vi "_computeInput.vi"(10 "HistoryYUR":dbl[][][](array[numeric]), 11 "Coeff.RST":dbl[][][](array[numeric])) -> (3 "u":dbl[](array[numeric]))   [LabVIEW 2021, in "System.lvclass"]
uses:
  System.lvclass
  <vilib>/Analysis/baseanly.llb/Real Dot Product.vi
  System.lvclass/System.ctl
  <vilib>/Analysis/NI_AALBase.lvlib
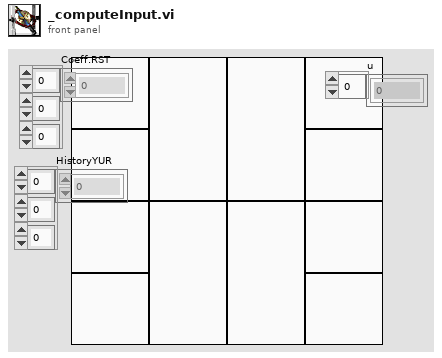
[diagram p1: front panel]
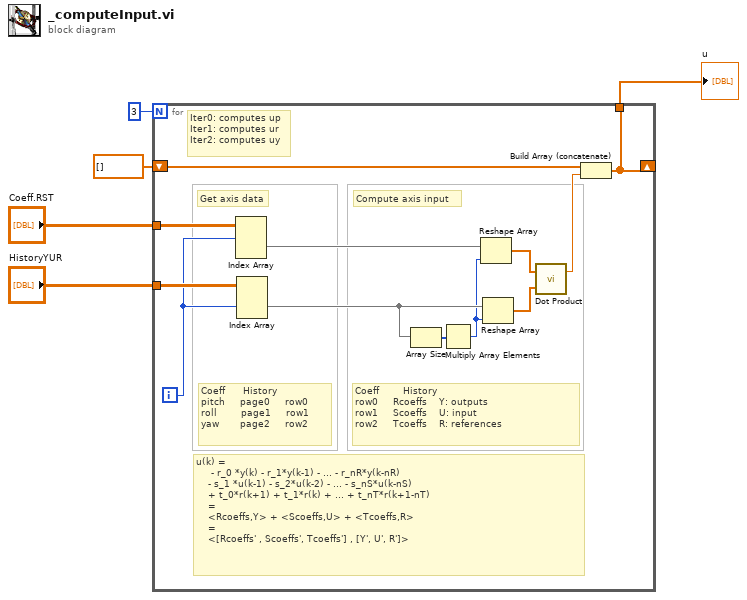
[diagram p0: block diagram]
diagram:
  n1 = for {
    N: 3 -> [_]
    tunnel: "Coeff.RST" -> [w17]
    tunnel: "HistoryYUR" -> [w16]
    shift-right: [w7] -> _
    shift-left: dbl[] [] -> [w8]
    tunnel: [w7] -> w5
    i -> [w6]
    # "u(k) = \n     - r_0 *y(k) - r_1*y(k-1) - ... - r_nR*y(k-nR) \n    - s_1 *u(k-1) - s_2*u(k-2) - ... - s_nS*u(k-nS) \n    + t_0*r(k+1) + t_1*r(k) + ... + t_nT*r(k+1-nT)\n    =\n    <Rcoeffs,Y> + <Scoeffs,U> + <Tcoeffs,R>\n    = \n    <[Rcoeffs' , Scoeffs', Tcoeffs'] , [Y', U', R']>"
    # "Iter0: computes up\nIter1: computes ur\nIter2: computes uy"
    # "Compute axis input"
    # "Coeff        History\nrow0     Rcoeffs    Y: outputs\nrow1     Scoeffs    U: input\nrow2     Tcoeffs    R: references"
    # "Get axis data"
    # "Coeff      History\npitch     page0     row0\nroll        page1     row1\nyaw       page2     row2"
    n2 = Index Array(array=w17, index (dim 0)=w6) -> (element=w15:dbl[][])  [unwired: 2 in]
    n3 = Index Array(array=w16, index (dim 1)=w6) -> (element=w13:dbl[][])  [unwired: 2 in]
    n4 = Array Size(array=w13) -> (size(s)=w14:i32[])
    n5 = Multiply Array Elements(1:w14) -> (0:w12:i32)
    n6 = Reshape Array(w15, w12) -> (w11:dbl[])
    n7 = Reshape Array(w13, w12) -> (w10:dbl[])
    n8 = call-poly <vilib>:"Dot Product.vi"("Y Vector"=w10, "X Vector"=w11) -> ("X * Y"=w9:dbl)  [unwired: 1 out]
    n9 = Build Array (concatenate)(w8, w9) -> (w7:dbl[])
  }
  "u" <- w5
